vi "parte_4.vi"(10 "array":i32[](array[numeric]), 11 "error_pin":i32) -> (3 "Boolean":bool)   [LabVIEW 2021]
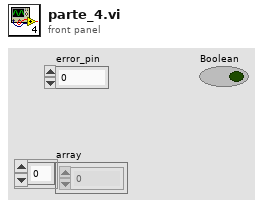
[diagram p1: front panel]
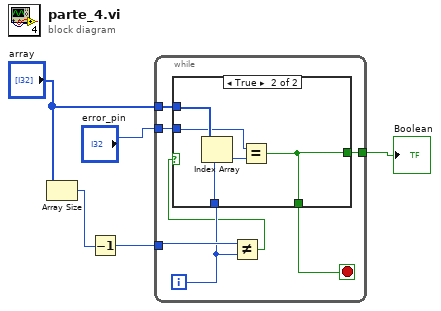
[diagram p0: block diagram]
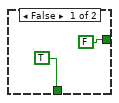
[diagram p2: hidden frame]
diagram:
  n1 = Array Size(array="array") -> (size(s)=w3:i32)
  n2 = Decrement(x=w3) -> (x-1=w4:i32)
  n3 = while {
    tunnel: "array" -> [w12]
    tunnel: "error_pin" -> [w11]
    tunnel: w4 -> [w10]
    tunnel: [w6] -> w1
    i -> [w9]
    stop <- w7 stop-if-true
    n4 = Not Equal?(x=w10, y=w9) -> (x != y?=w8:bool)
    n5 = case shown="True" w8 {
      tunnel: w12 -> [_ w19]
      tunnel: w11 -> [_ w18]
      tunnel: w9 -> [_ w16]
      tunnel: [TRUE w15] -> w7
      tunnel: [FALSE w15] -> w6
      frame False {
      }
      frame True {
        n6 = Index Array(array=w19, index=w16) -> (element=w17:i32)
        n7 = Equal?(x=w18, y=w17) -> (x = y?=w15:bool)
      }
    }
  }
  "Boolean" <- w1
